vi "AddCircle.vi"(4 "centerY":dbl, 6 "centerX":dbl, 9 "radius":dbl=34.0, 10 "vertical":dbl[](array[numeric]), 11 "horizontal":dbl[](array[numeric])) -> (3 "output":cluster{"horizontal":dbl[], "vertical":dbl[]}[](array[cluster]))   [LabVIEW 2014]
uses:
  <vilib>/imath/engines/lvmath2/RunTimeEngine/RangeToken/NIMS_Range.vi
  <instcachedir>/0/NIMS_Range_9BCE657718DF4976A877346C61F22738.lvgen/NIMS_Range_9BCE657718DF4976A877346C61F22738_000.vi
  <vilib>/imathl/engines/lvmath/Functions/Error Handling/Create Error.vi
  <vilib>/imath/engines/lvmath2/RunTimeEngine/NodeEndStatement/NIMS_NodeEndStatement_Output.vi
  <instcachedir>/0/NIMS_NodeEndStatement_Output_53EC0D466D134D7ABD903AC30B43404B.lvgen/NIMS_NodeEndStatement_Output_53EC0D466D134D7ABD903AC30B43404B_005.vi
  <vilib>/imath/engines/lvmath2/RunTimeEngine/ErrorHandling/NIMS_Finalize Error.vi
panel:
  out "x":dbl[](array[numeric])
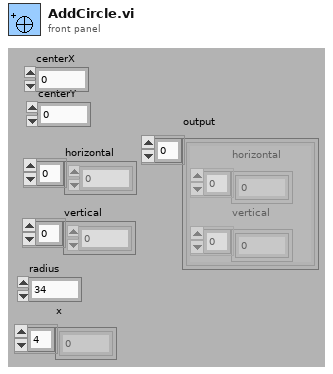
[diagram p1: front panel]
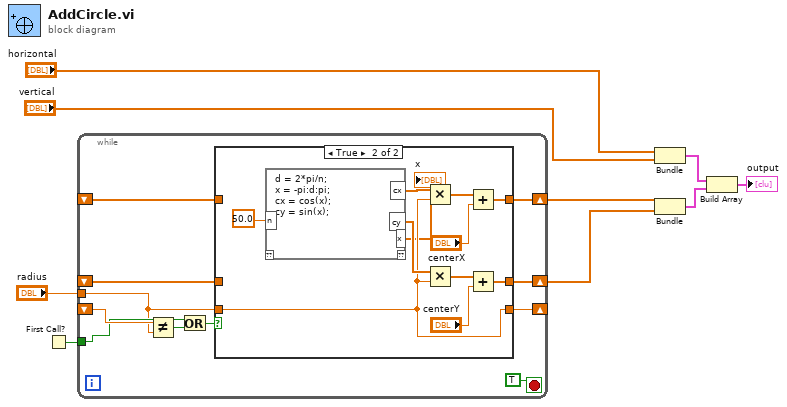
[diagram p0: block diagram]
diagram:
  n1 = First Call?() -> (First Call?: T/F=w7:bool)
  n2 = while {
    shift-right: [w19] -> w9
    shift-left: _ -> [w17]
    shift-right: [w18] -> w8
    shift-left: _ -> [w16]
    shift-right: [w15] -> _
    shift-left: _ -> [w14]
    tunnel: w7 -> [w11]
    tunnel: "radius" -> [w10]
    stop <- TRUE stop-if-true
    n3 = Not Equal?(x=w14, y=w10) -> (x != y?=w13:bool)
    n4 = Or(x=w11, y=w13) -> (x .or. y?=w12:bool)
    n5 = case shown="True" w12 {
      tunnel: [w23 w27] -> w19
      tunnel: [w22 w26] -> w18
      tunnel: w17 -> [w23 _]
      tunnel: w16 -> [w22 _]
      tunnel: w10 -> [w21 w25]
      tunnel: [w21 w25] -> w15
      frame False {
      }
      frame True {
        n6 = mathscript code="d = 2*pi/n;\nx = -pi:d:pi;\ncx = cos(x);\ncy = sin(x);"("n"=50.0) -> ("cx"=w29:dbl[], "cy"=w28:dbl[], "x"=→"x":dbl[])  [unwired: 1 in, 1 out]
        n7 = Multiply(x=w29, y=w25) -> (x*y=w34:dbl[])
        n8 = Multiply(x=w28, y=w25) -> (x*y=w33:dbl[])
        n9 = Add(x=w34, y="centerX") -> (x+y=w27:dbl[])
        n10 = Add(x=w33, y="centerY") -> (x+y=w26:dbl[])
      }
    }
  }
  n11 = Bundle("horizontal"="horizontal", "vertical"="vertical") -> (w4:cluster{"horizontal":dbl[], "vertical":dbl[]})  [unwired: 1 in]
  n12 = Bundle(w9, w8) -> (w3:cluster{dbl[], dbl[]})  [unwired: 1 in]
  n13 = Build Array(w4, w3) -> (→"output":cluster{"horizontal":dbl[], "vertical":dbl[]}[])
